vi "Unicode Write Text File Example.vi"() -> ()   [LabVIEW 2020]
doc: "This example demonstrates writing unicode text to a file."
uses:
  Unicode/Controls/String Encoding.ctl
  Types/Encoded UTF-8 String.ctl
  Types/UTF-8 String/UTF-8 String.lvclass/UTF-8 String.ctl
  Types/UTF-8 Path/UTF-8 Path.lvclass/UTF-8 Path.ctl
  1bf067af-972d-466b-9d68-d02e2bdd837e.vi
  94f2b1b0-f483-4077-9deb-c3828a516b03.vi
  7815f275-58e2-44b2-80c9-6b9e48860ffb.vi
  c100b62a-dfcd-489d-b2f4-78549eda4701.vi
  Unicode/Encode String.vi
  Private/Conversion/Path as UTF-8 Path.vi
  Private/Conversion/Polymorphic VIs/Path as UTF-8 Path (UTF-8 Path).vi
  1bf067af-972d-466b-9d68-d02e2bdd837e.vi/8b166e89-7f88-4d33-9f65-0e5b55cfdfba.vi
  1bf067af-972d-466b-9d68-d02e2bdd837e.vi/154c5264-acfe-4024-9e59-4207c26e417f.vi
  1bf067af-972d-466b-9d68-d02e2bdd837e.vi/a2237eed-bac6-4067-93fc-b5fa504ea8ff.vi
  <vilib>/Utility/error.llb/Clear Errors.vi
  1bf067af-972d-466b-9d68-d02e2bdd837e.vi/5e3a38b3-3d0f-4559-ad1c-eed73d89bfdc.vi
  1bf067af-972d-466b-9d68-d02e2bdd837e.vi/c6c6a2d4-2ed2-47c1-bb47-bf9afb14d634.vi
  1bf067af-972d-466b-9d68-d02e2bdd837e.vi/07ae02c5-2d8e-47e7-881c-96fbd466826f.vi
  1bf067af-972d-466b-9d68-d02e2bdd837e.vi/7af25b42-1b06-4de4-a75a-8ed1001daaff.vi
  1bf067af-972d-466b-9d68-d02e2bdd837e.vi/e07117c9-d87a-4df6-978c-25aa8b1cd0ee.vi
  Types/UTF-8 String/Write Encoded UTF-8 String.vi
  Private/Conversion/String as Encoded String.vi
  Private/Conversion/Polymorphic VIs/String as Encoded String (UTF-8 String).vi
  File IO/Short Name to Path (Unicode).vi
  Types/UTF-8 Path/New UTF-8 Path.vi
  c100b62a-dfcd-489d-b2f4-78549eda4701.vi/cd814f09-858d-41ec-a1ea-d598fdb95b0d.vi
  c100b62a-dfcd-489d-b2f4-78549eda4701.vi/cdde7a24-321d-4ebe-8fa8-ef041a4f6d83.vi
  Private/Conversion/Text as Encoded String.vi
  Private/Conversion/Polymorphic VIs/Text as Encoded String (UTF-8 Path).vi
  Private/Library/gu_delete.vi
  c100b62a-dfcd-489d-b2f4-78549eda4701.vi/80924ba4-6f01-46cb-bebd-728ad922c70d.vi
  Private/Conversion/String as UTF-8 String.vi
  Private/Conversion/Polymorphic VIs/String as UTF-8 String (UTF-8 String).vi
  Unicode/Detect String Encoding.vi
  Private/Conversion/Text to UTF-8.vi
  Private/Conversion/Polymorphic VIs/Text to UTF-8 (LabVIEW String).vi
  Private/Conversion/Encoded UTF-8 String to Encoded UTF-16LE String.vi
  Unicode/SubVIs/UTF-16 Byte Swap.vi
  Private/Conversion/UTF-8 to Text.vi
  Private/Conversion/Polymorphic VIs/UTF-8 to Text (LabVIEW String).vi
  Private/Conversion/Encoded UTF-16LE String to Encoded UTF-8 String.vi
  Unicode/Prepend BOM.vi
  Private/Conversion/Polymorphic VIs/String as Encoded String (LabVIEW String).vi
  Private/Library/gu_open_file_dialog.vi
  Private/Library/gu_select_folder_dialog.vi
  Types/UTF-8 Path/Write Encoded UTF-8 Path.vi
  Private/Library/gu_create_file.vi
  1bf067af-972d-466b-9d68-d02e2bdd837e.vi/07ae02c5-2d8e-47e7-881c-96fbd466826f.vi/b0de225b-b813-4a3f-91fa-b2c78c384815.vi
  1bf067af-972d-466b-9d68-d02e2bdd837e.vi/07ae02c5-2d8e-47e7-881c-96fbd466826f.vi/b1dd94da-e188-4359-85d0-d6693b26af46.vi
  1bf067af-972d-466b-9d68-d02e2bdd837e.vi/07ae02c5-2d8e-47e7-881c-96fbd466826f.vi/2799960a-efad-449d-b375-cc5363f1c370.vi
  1bf067af-972d-466b-9d68-d02e2bdd837e.vi/07ae02c5-2d8e-47e7-881c-96fbd466826f.vi/2ed7adf8-1da0-426c-b32d-a1b4538e7e16.vi
  Private/Conversion/Text as String.vi
  Private/Conversion/Polymorphic VIs/Text as String (UTF-8 Path).vi
  Types/UTF-8 String/Read Encoded UTF-8 String.vi
  Private/Library/gu_long_path.vi
  Types/UTF-8 Path/Read Encoded UTF-8 Path.vi
  Private/Library/Result To Error.vi
  Private/Conversion/Polymorphic VIs/Text as String (UTF-8 String).vi
  Unicode/Strip BOM.vi
  Unicode/Detect String Encoding.vi/f4e2713d-ca87-487a-b901-d606fc3002c3.vi
  Unicode/SubVIs/Byte Order Marks.vi
  Unicode/Detect BOM.vi
  Private/Memory/Copy String.vi
  Private/Memory/Copy String.vi/4d47babd-4a2d-4eb7-b91b-7e707d692665.vi
  Private/Library/gu_free.vi
  Private/Library/gu_is_text_utf16.vi
  Private/Library/gu_is_text_utf8.vi
  <vilib>/Utility/error.llb/Error Cluster From Error Code.vi
  Private/Memory/Copy String Array.vi
  Private/Library/gu_message_box.vi
  Types/UTF-8 String/UTF-8 String.lvclass
  Types/UTF-8 Path/UTF-8 Path.lvclass
  G-Unicode.lvlib
panel:
  in  "Delete File Afterwards":bool=TRUE
  in  "Output File Encoding":T1=enum."UTF-8"
  # "Instructions:\n1. Select an encoding to save the file in Output File Encoding, and whether the example file should be deleted afterwards, then run the VI.\n2. Select a file path to save the text file.\n3. Example unicode text will be converted to the selected encoding and saved to the file.\n4. Notepad will be automatically opened to display the new file.\n5. Confirm the file encoding in the lower right of the Notepad window.\n6. Close Notepad."
  # "G"
  # "-Unicode"
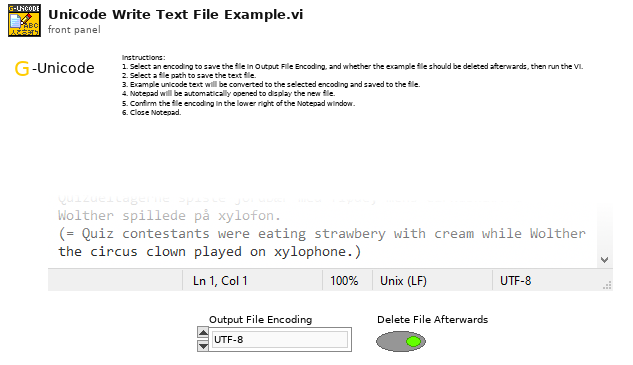
[diagram p1: front panel]
types:
  T1 = typedef "G-Unicode.lvlib/String Encoding.ctl" = enum16{"ANSI", "UTF-8", "UTF-16LE", "UTF-16BE", "Unknown"}
  T2 = enum16{"open", "replace", "create", "open or create", "replace or create", "replace or create with confirmation"}
  T3 = typedef "G-Unicode.lvlib/Encoded UTF-8 String.ctl" = string
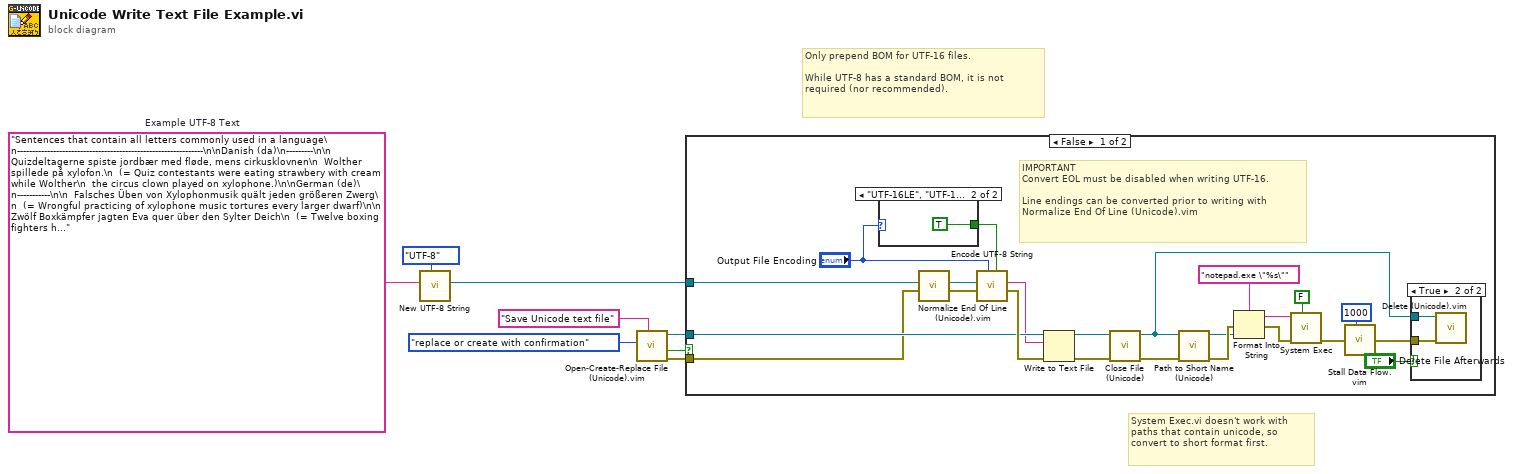
[diagram p0: block diagram]
diagram:
  w8 = T3 "Sentences that contain all letters commonly used in a language\n--------------------------------------------------------------\n\nDanish (da)\n---------\n\n  Quizdeltagerne spiste jordbær med fløde, mens cirkusklovnen\n  Wolther spillede på xylofon.\n  (= Quiz contestants were eating strawbery with cream while Wolther\n  the circus clown played on xylophone.)\n\nGerman (de)\n-----------\n\n  Falsches Üben von Xylophonmusik quält jeden größeren Zwerg\n  (= Wrongful practicing of xylophone music tortures every larger dwarf)\n\n  Zwölf Boxkämpfer jagten Eva quer über den Sylter Deich\n  (= Twelve boxing fighters hunted Eva across the dike of Sylt)\n\n  Heizölrückstoßabdämpfung\n  (= fuel oil recoil absorber)\n  (jqvwxy missing, but all non-ASCII letters in one word)\n\nEnglish (en)\n------------\n\n  The quick brown fox jumps over the lazy dog\n\nSpanish (es)\n------------\n\n  El pingüino Wenceslao hizo kilómetros bajo exhaustiva lluvia y \n  frío, añoraba a su querido cachorro.\n  (Contains every letter and every accent, but not every combination\n  of vowel + acute.)\n\nFrench (fr)\n-----------\n\n  Portez ce vieux whisky au juge blond qui fume sur son île intérieure, à\n  côté de l'alcôve ovoïde, où les bûches se consument dans l'âtre, ce\n  qui lui permet de penser à la cænogenèse de l'être dont il est question\n  dans la cause ambiguë entendue à Moÿ, dans un capharnaüm qui,\n  pense-t-il, diminue çà et là la qualité de son œuvre. \n\n  l'île exiguë\n  Où l'obèse jury mûr\n  Fête l'haï volapük,\n  Âne ex aéquo au whist,\n  Ôtez ce vœu déçu.\n\n  Le cœur déçu mais l'âme plutôt naïve, Louÿs rêva de crapaüter en\n  canoë au delà des îles, près du mälström où brûlent les novæ.\n\nIrish Gaelic (ga)\n-----------------\n\n  D'fhuascail Íosa, Úrmhac na hÓighe Beannaithe, pór Éava agus Ádhaimh\n\nHungarian (hu)\n--------------\n\n  Árvíztűrő tükörfúrógép\n  (= flood-proof mirror-drilling machine, only all non-ASCII letters)\n\nIcelandic (is)\n--------------\n\n  Kæmi ný öxi hér ykist þjófum nú bæði víl og ádrepa\n\n  Sævör grét áðan því úlpan var ónýt\n  (some ASCII letters missing)\n\nJapanese (jp)\n-------------\n\n  Hiragana: (Iroha)\n\n  いろはにほへとちりぬるを\n  わかよたれそつねならむ\n  うゐのおくやまけふこえて\n  あさきゆめみしゑひもせす\n\n  Katakana:\n\n  イロハニホヘト チリヌルヲ ワカヨタレソ ツネナラム\n  ウヰノオクヤマ ケフコエテ アサキユメミシ ヱヒモセスン\n\nHebrew (iw)\n-----------\n\n  ? דג סקרן שט בים מאוכזב ולפתע מצא לו חברה איך הקליטה\n\nPolish (pl)\n-----------\n\n  Pchnąć w tę łódź jeża lub ośm skrzyń fig\n  (= To push a hedgehog or eight bins of figs in this boat)\n\nRussian (ru)\n------------\n\n  В чащах юга жил бы цитрус? Да, но фальшивый экземпляр!\n  (= Would a citrus live in the bushes of south? Yes, but only a fake one!)\n\nThai (th)\n---------\n\n  [--------------------------|------------------------]\n  ๏ เป็นมนุษย์สุดประเสริฐเลิศคุณค่า  กว่าบรรดาฝูงสัตว์เดรัจฉาน\n  จงฝ่าฟันพัฒนาวิชาการ           อย่าล้างผลาญฤๅเข่นฆ่าบีฑาใคร\n  ไม่ถือโทษโกรธแช่งซัดฮึดฮัดด่า     หัดอภัยเหมือนกีฬาอัชฌาสัย\n  ปฏิบัติประพฤติกฎกำหนดใจ        พูดจาให้จ๊ะๆ จ๋าๆ น่าฟังเอย ฯ\n\n  [The copyright for the Thai example is owned by The Computer\n  Association of Thailand under the Royal Patronage of His Majesty the\n  King.]\n"  # Example UTF-8 Text
  # "System Exec.vi doesn't work with paths that contain unicode, so convert to short format first."
  # "Only prepend BOM for UTF-16 files.\n\nWhile UTF-8 has a standard BOM, it is not required (nor recommended)."
  n1 = call "New UTF-8 String.vi"("Input Encoding (ANSI)"=String_Encoding."UTF-8", "String"=w8) -> ("UTF-8 String"=w4:refnum<class "UTF-8 String.lvclass">)  [unwired: 8 in, 1 out]
  n2 = call "Open-Create-Replace File (Unicode).vim"("Prompt"="Save Unicode text file", "Operation (0:open)"=T2."replace or create with confirmation") -> ("error out"=w1:errorcluster, "Cancelled"=w2:bool, "Refnum out"=w3:refnum<file>)  [unwired: 7 in]
  n3 = case shown="False" w2 {
    tunnel: w4 -> [w11 _]
    tunnel: w3 -> [w21 _]
    tunnel: w1 -> [w10 _]
    frame False {
      # "IMPORTANT\nConvert EOL must be disabled when writing UTF-16.\n\nLine endings can be converted prior to writing with Normalize End Of Line (Unicode).vim"
      n4 = case shown="\"UTF-16LE\", \"UTF-16BE\"" "Output File Encoding" {
        tunnel: [_ TRUE] -> w31
        frame Default {
        }
        frame "UTF-16LE", "UTF-16BE" {
        }
      }
      n5 = call "Normalize End Of Line (Unicode).vim"("String"=w11, "error in"=w10) -> ("Normalized String"=w12:refnum<class "UTF-8 String.lvclass">, "error out"=w9:errorcluster)  [unwired: 7 in]
      n6 = call "Encode UTF-8 String.vi"("Prepend BOM (F)"=w31, "Output Encoding (UTF-16LE)"="Output File Encoding", "error in (no error)"=w9, "UTF-8 String"=w12) -> ("error out"=w27:errorcluster, "Encoded String"=w20:string)  [unwired: 6 in]
      n7 = Write to Text File(file (use dialog)=w21, text=w20, error in=w27) -> (refnum out=w29:refnum<file>, error out=w28:errorcluster)  [unwired: 1 in, 1 out]
      n8 = call "Close File (Unicode).vi"("error in"=w28, "Refnum"=w29) -> ("error out"=w18:errorcluster, "UTF-8 Path"=w19:refnum<class "UTF-8 Path.lvclass">)  [unwired: 8 in]
      n9 = call "Path to Short Name (Unicode).vi"("error in"=w18, "Path"=w19) -> ("error out"=w17:errorcluster, "LabVIEW Path"=w16:path)  [unwired: 8 in]
      n10 = Format Into String(format string="notepad.exe \"%s\"", error in=w17, w16) -> (resulting string=w26:string, error out=w24:errorcluster)  [unwired: 1 in]
      n11 = call <vilib>:"System Exec.vi"("wait until completion? (T)"=FALSE, "error in (no error)"=w24, "command line"=w26) -> ("error out"=w23:errorcluster)  [unwired: 5 in, 3 out]
      n12 = call "Stall Data Flow.vim"("value in"=w23, "milliseconds to wait"=u32 1000) -> ("value out"=w14:errorcluster)  [unwired: 1 out]
      n13 = case shown="True" "Delete File Afterwards" {
        tunnel: w14 -> [_ w33]
        tunnel: w19 -> [_ w32]
        frame False {
        }
        frame True {
          n14 = call "Delete (Unicode).vim"("error in"=w33, "Path"=w32) -> ()  [unwired: 7 in, 3 out]
        }
      }
    }
    frame True {
    }
  }
